vi "FPGA_TEST_microStepLoop.vi"(8 "Clock Trigger":bool, 9 "ResetUstep":bool, 10 "CorrectedIncrement":i32, 11 "StepsInAramp":i32) -> (0 "MaxPulse":bool, 1 "BotRamp":bool, 2 "NextUstep":i32, 3 "CurrentUstep":i32)   [LabVIEW 2016]
uses:
  <vilib>/Platform/TimedLoop/XDataNode/timing_clust.ctl
  <vilib>/Platform/TimedLoop/XDataNode/nitl_modes.ctl
  <vilib>/Platform/TimedLoop/XDataNode/wakeup.ctl
  <vilib>/rvi/Emulation/niFpgaSctlEmulationGetInTimedLoop.vi
  <vilib>/rvi/Emulation/niFpgaEmulationReportErrorSimple.vi
  <vilib>/rvi/Emulation/niFpgaGetClockAttributes.vi
  <vilib>/rvi/Emulation/niFpgaCriticalErrorInLSC.vi
  <vilib>/Platform/TimedLoop/XDataNode/XDataNode.xnode
  <vilib>/Platform/TimedLoop/XDataNode/XDNodeRunTimeDep.lvlib
panel:
  out "TopRamp":bool
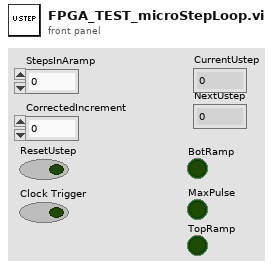
[diagram p1: front panel]
types:
  T1 = typedef "XDNodeRunTimeDep.lvlib/timing_clust.ctl" = cluster{"Expected End [f-1]":u64, "Actual End [f-1]":u64, "Finished Late? [f-1]":bool, "Expected End [i-1]":u64, "Actual End [i-1]":u64, "Finished Late? [i-1]":bool, "Expected Start [i]":u64, "Actual Start [i]":u64, "Expected Start [f]":u64, "Actual Start [f]":u64, "Source Name":string, "Structure Name":string, "Period":i64, "Deadline":i64, "Offset":i64, "Start":i64, "Priority":i32, "Timeout":i32, "Mode":T2, "Wakeup Reason":T3, "Error":errorcluster, "Source Type":string, "Secondary Source Type":string, "Global End Time":u64, "Global Start Time":u64, "Frame Duration":u64, "Iteration Duration":u64, "Assigned CPU":i32, "I/O Scan Engine Mode":u32}
  T2 = typedef "XDNodeRunTimeDep.lvlib/nitl_modes.ctl" = enum32{"No Change", "Process missed periods, maintain original phase", "Discard missed periods, maintain original phase", "Process missed periods, ignore original phase", "Discard missed periods, ignore original phase"}
  T3 = typedef "XDNodeRunTimeDep.lvlib/wakeup.ctl" = enum32{"Normal", "Aborted", "Asynchronous wakeup", "Timing source error", "Timed loop error", "Timeout"}
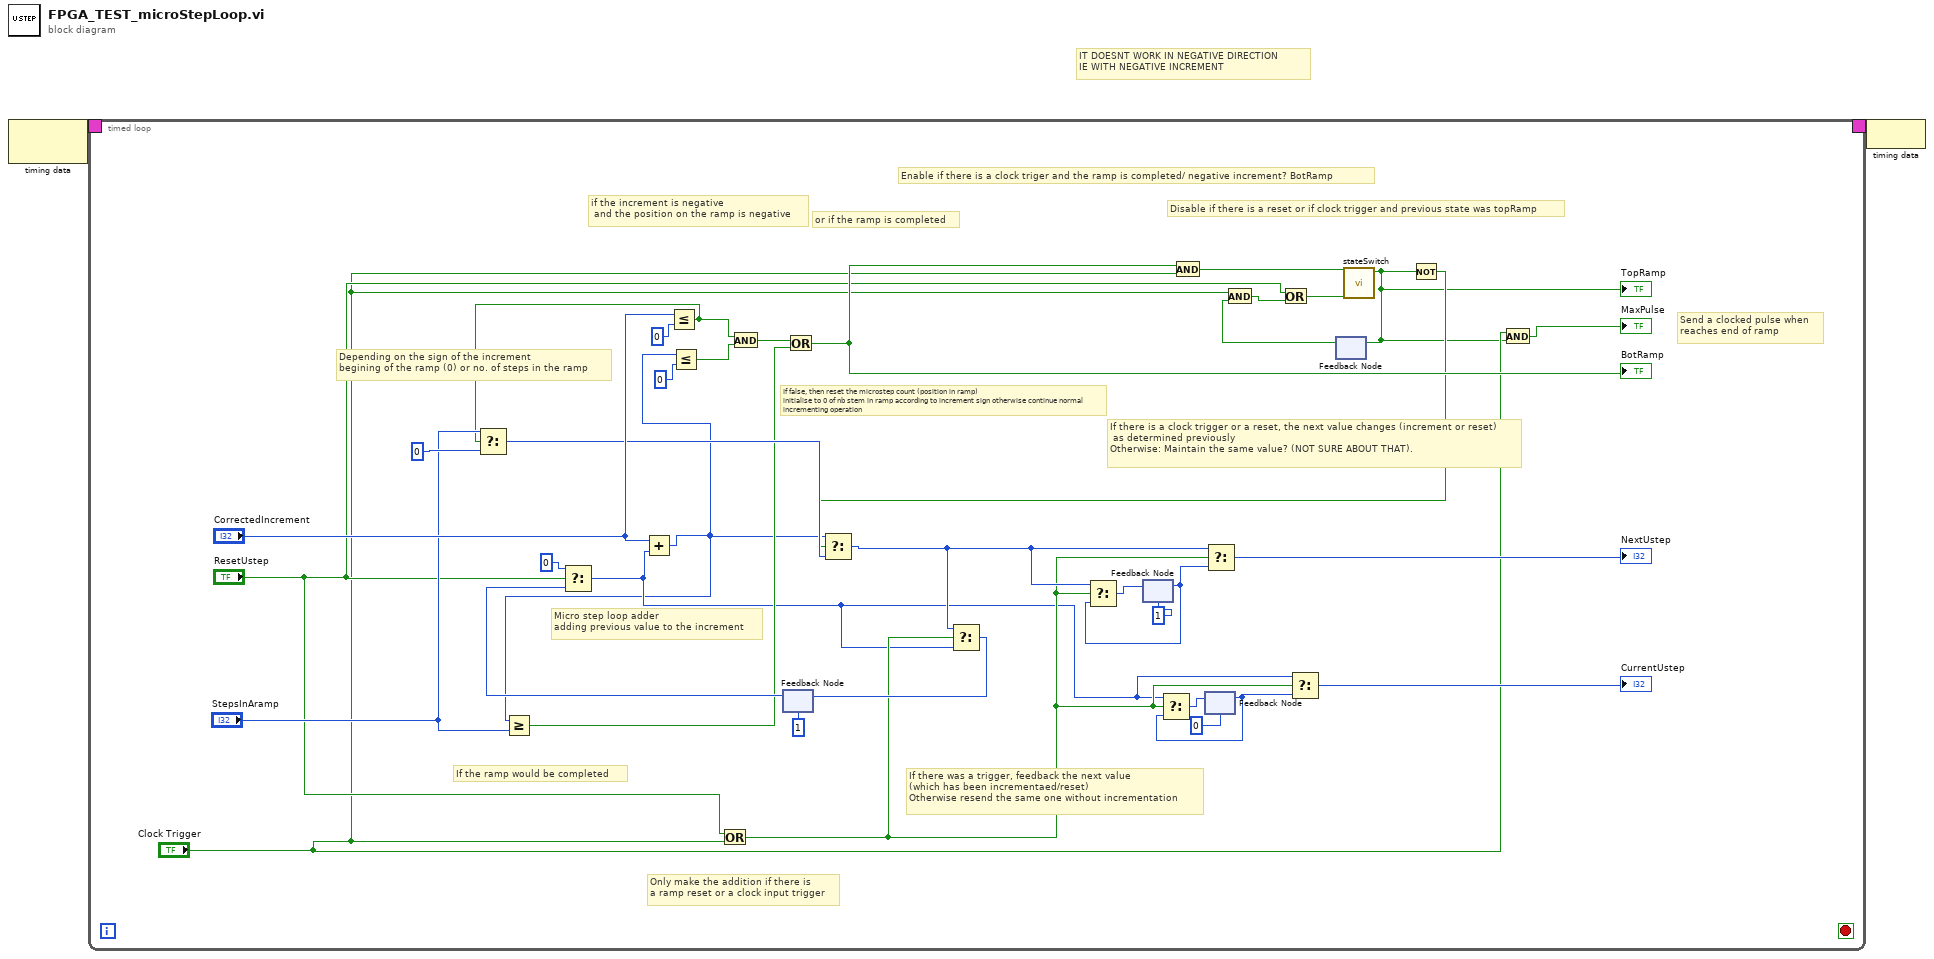
[diagram p0: block diagram]
diagram:
  # "IT DOESNT WORK IN NEGATIVE DIRECTION\nIE WITH NEGATIVE INCREMENT"
  n1 = node-c288() -> (w2:T1)  [unwired: 1 in]
  n2 = timed-loop {
    timing: w2 -> [_]
    timing-out: [_] -> w1
    stop <- _ stop-if-true
    # "Disable if there is a reset or if clock trigger and previous state was topRamp"
    # "Enable if there is a clock triger and the ramp is completed/ negative increment? BotRamp"
    # "or if the ramp is completed"
    # "If there was a trigger, feedback the next value \n(which has been incrementaed/reset)\nOtherwise resend the same one without incrementation"
    # "If there is a clock trigger or a reset, the next value changes (increment or reset)\n as determined previously\nOtherwise: Maintain the same value? (NOT SURE ABOUT THAT)."
    # "If false, then reset the microstep count (position in ramp)\ninitialise to 0 of nb stem in ramp according to increment sign otherwise continue normal incrementing operation"
    # "Depending on the sign of the increment\nbegining of the ramp (0) or no. of steps in the ramp"
    # "if the increment is negative \n and the position on the ramp is negative"
    # "Only make the addition if there is\na ramp reset or a clock input trigger"
    # "Send a clocked pulse when\nreaches end of ramp"
    # "Micro step loop adder\nadding previous value to the increment"
    # "If the ramp would be completed"
    n3 = Less Or Equal?(x="CorrectedIncrement", y=0) -> (x <= y?=w28:bool)
    n4 = Select(t="StepsInAramp", s=w28, f=0) -> (s? t:f=w27:i32)
    n5 = Or(x="ResetUstep", y="Clock Trigger") -> (x .or. y?=w14:bool)
    n6 = feedback #1(1) -> (w36:i32)
    n7 = Select(t=0, s="ResetUstep", f=w36) -> (s? t:f=w4:i32)
    n8 = Add(x="CorrectedIncrement", y=w4) -> (x+y=w3:i32)
    n9 = Greater Or Equal?(x=w3, y="StepsInAramp") -> (x >= y?=w19:bool)
    n10 = Less Or Equal?(x=w3, y=0) -> (x <= y?=w31:bool)
    n11 = And(x=w28, y=w31) -> (x .and. y?=w20:bool)
    n12 = Or(x=w20, y=w19) -> (x .or. y?=w13:bool)
    "BotRamp" <- w13
    n13 = feedback #2(1) -> (w24:i32)
    n14 = And(x=w13, y="Clock Trigger") -> (x .and. y?=w12:bool)
    n15 = feedback #3(0 ("t")) -> (w17:i32)
    n16 = Select(t=w4, s=w14, f=w17) -> (s? t:f=w18:i32)
    n17 = feedback-in #3(w18) -> ()
    n18 = Select(t=w4, s=w14, f=w17) -> (s? t:f=→"CurrentUstep":i32)
    n19 = feedback #4() -> (w5:bool)  [unwired: 1 in]
    n20 = And(x="Clock Trigger", y=w5) -> (x .and. y?=w10:bool)
    n21 = Or(x="ResetUstep", y=w10) -> (x .or. y?=w11:bool)
    n22 = call "stateSwitch.vi"("disable"=w11, "enable"=w12) -> ("state"=w6:bool)  [unwired: 9 in]
    "TopRamp" <- w6
    n23 = feedback-in #4(w6) -> ()
    n24 = Not(x=w6) -> (.not. x?=w7:bool)
    n25 = Select(t=w3, s=w7, f=w27) -> (s? t:f=w22:i32)
    n26 = Select(t=w22, s=w14, f=w4) -> (s? t:f=w21:i32)
    n27 = feedback-in #1(w21) -> ()
    n28 = Select(t=w22, s=w14, f=w24) -> (s? t:f=w25:i32)
    n29 = feedback-in #2(w25) -> ()
    n30 = Select(t=w22, s=w14, f=w24) -> (s? t:f=→"NextUstep":i32)
    n31 = And(x="Clock Trigger", y=w6) -> (x .and. y?=→"MaxPulse":bool)
  }
  n32 = node-c288(w1) -> ()
